vi "Scope_5761.vi"() -> ()   [LabVIEW 2013]
uses:
  <vilib>/userdefined/High Color/nirio_resource_hc.ctl
  FPGA/DataMode.ctl
  <vilib>/Analysis/4window.llb/windowTd.ctl
  Host/Scope/controls/power_spectrum_unit.ctl
  Host/Scope5782/Scope/controls/5782_trigger_type.ctl
  Host/Scope/controls/Data_calc_mode.ctl
  Host/Scope/controls/Data_display_mode.ctl
  Host/Scope/controls/Graph_references.ctl
  Host/Scope/controls/graph_controls.ctl
  Host/Scope/controls/Channel_select.ctl
  Host/Communication/Driver/RemoteConnection/RemoteConnection.lvclass
  Host/FpgaRef/FpgaRef5761/ClockSource_5761.ctl
  Host/Scope/Scope5671/Scope5761.lvclass
  Host/Scope/ScopeBase/ScopeBase.lvclass/ScopeBase.ctl
  FPGA/fpga_settings.ctl
  Host/Scope/controls/ScopeMode.ctl
  Host/Communication/global_stop.vi
  <vilib>/FPGAPlugInAG/PXIe-7975R/niLvFpga_Open_PXIe-7975R.vi
  <vilib>/rvi/interface/common/dynamic/niFpgaDynamicAddResources.vi
  <vilib>/rvi/interface/nirviOpenFPGA/nirviOpenFPGA.xnode
  FPGA Bitfiles/FPGAmain_5761_zPCTJJmozx4.lvbitx
  FPGAmain_5761.vi
  FPGA Bitfiles/FPGAmain5782_W462Q9ePIkg.lvbitx
  <vilib>/rvi/FXPMathLib/FxpInterpret/XNode/nifxpmath_Interpret.xnode
  Host/FpgaRef/FpgaRef5761/FpgaRef5761.lvclass
  Host/Scope/ScopeBase/ScopeBase.lvclass
  Host/FpgaRef/FpgaRef5782/FpgaRef5782.lvclass
  <vilib>/Analysis/NI_AALPro.lvlib
panel:
  in  "5761 -1  resource 2":T1="RIO0"
  in  "5761 -1  resource":T1="RIO0"
  in  "Ch3":bool
  in  "Ch2":bool
  in  "Ch1":bool
  in  "Ch0":bool
  in  "Ch3":bool
  in  "Ch2":bool
  in  "Ch1":bool
  in  "Ch0":bool
  in  "Ch3 Q":bool
  in  "Ch3 I":bool
  in  "Ch2 Q":bool
  in  "Ch2 I":bool
  in  "Ch1 Q":bool
  in  "Ch1 I":bool
  in  "Ch0 Q":bool
  in  "Ch0 I":bool
  in  "Ch3 Q":bool
  in  "Ch3 I":bool
  in  "Ch2 Q":bool
  in  "Ch2 I":bool
  in  "Ch1 Q":bool
  in  "Ch1 I":bool
  in  "Ch0 Q":bool
  in  "Ch0 I":bool
  in  "deltaF":bool
  in  "#bins":i32=1 min=1 max=16
  in  "ch1 DC offset":dbl caption="DC offset\nChannel 1"
  in  "ch0 DC offset":dbl caption="DC offset\nChannel 0"
  in  "Chart length":i32=200000
  in  "Trigmode":enum32{"Triggered", "Continuous"}(radio)
  in  "Refence for phase":T2
  in  "Graph_refs":T3
  out "Lower chart":dbl[][](graph)
  out "Upper chart":dbl[][](graph)
  out "Lower graph":i16[][](graph)
  in  "Buffer":T5
  in  "Display":T6
  in  "Trigger":T7
  in  "Ch1 Q":bool
  in  "Ch1 I":bool
  in  "Ch0 Q":bool
  in  "Ch0 I":bool
  in  "Ch1":bool
  in  "Ch0":bool
  out "stop 2":bool
  in  "Zoom freq X":bool
  in  "Zoom freq Y":bool
  in  "Zoom time Y":bool
  in  "Zoom time X":bool
  in  "Unit":T8
  in  "Window":T9=1 items=["Rectangle"=0, "Hanning"=1, "Hamming"=2, "Blackman-Harris"=3, "Exact Blackman"=4, "Blackman"=5, "Flat Top"=6, "4 Term B-Harris "=7, "7 Term B-Harris"=8, "Low Sidelobe"=9, "Blackman Nuttall"=11, "Triangle"=30, "Bartlett-Hanning"=31, "Bohman"=32, "Parzen"=33, "Welch"=34, "Kaiser"=60, "Dolph-Chebyshev"=61, "Gaussian"=62]
  in  "Samples per 5782 record":i32
  in  "Phase offset (deg)":dbl
  in  "Fequency [MHz]":dbl format="%#_8g"
  in  "Mode":T10
  in  "Mixer freq [MHz]":dbl
  out "freqdata":cluster{"f0":dbl, "df":dbl, "magnitude":dbl[]}[](graph)
  in  "Rumode":bool
  in  "Singleshot":bool
  out "error IO":errorcluster
  in  "stop":bool
  in  "resource name":T1="RIO0"
  # "5161 - 1"
  # "5161 - 2"
  # "FPGA setup"
  # "V"
  # "V"
  # "Auto Zoom"
  # "5782"
  # "5161 - 1"
  # "Simulated data"
  # "5161 - 2"
  # "FFT"
  # "Auto Zoom"
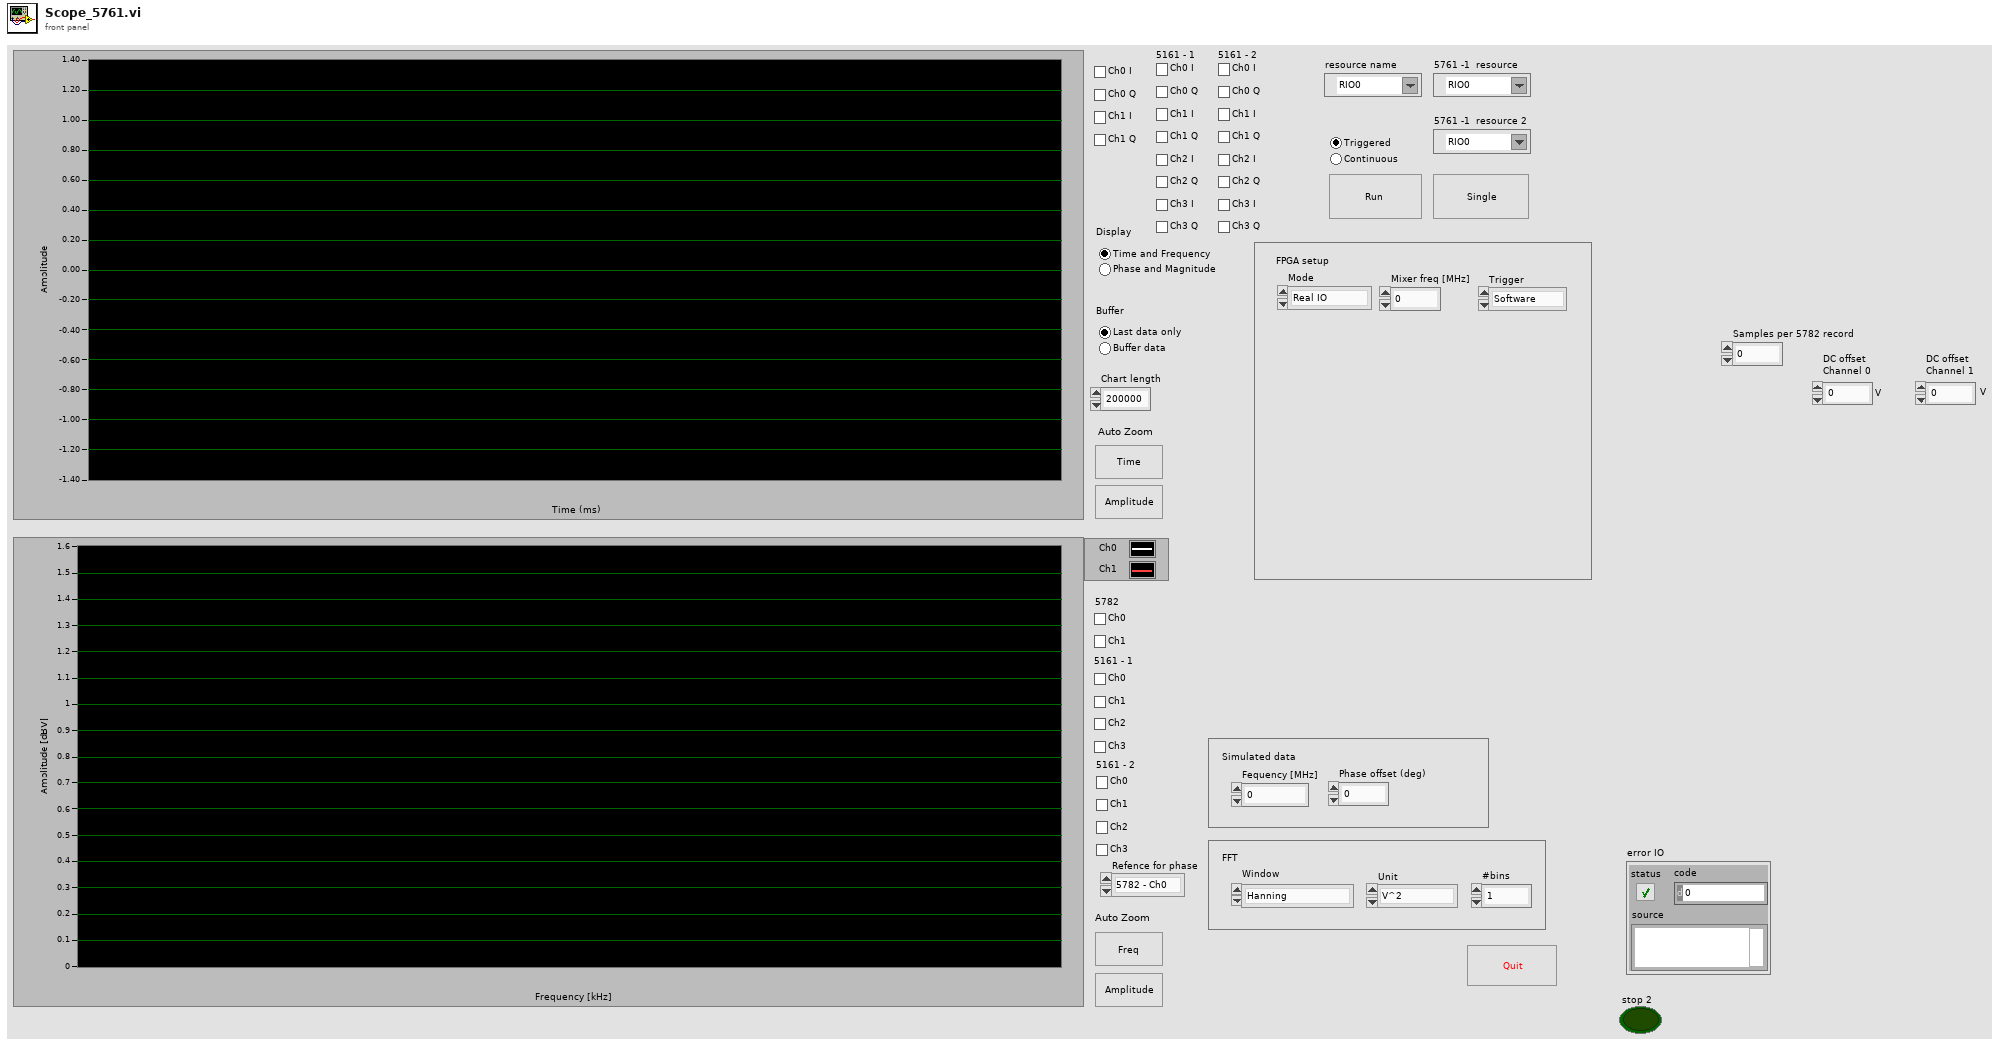
[diagram p1: front panel]
types:
  T1 = typedef "nirio_resource_hc.ctl" = tag
  T2 = typedef "Channel_select.ctl" = enum16{"5782 - Ch0", "5782 - Ch1"}
  T3 = typedef "Graph_references.ctl" = cluster{"upper":T4, "lower":T4, "Freq graph":refnum<vi>}
  T4 = typedef "graph_controls.ctl" = cluster{"Graph":refnum<vi>, "Time btn":refnum<vi>, "Amplitude btn":refnum<vi>, "Chart":refnum<vi>}
  T5 = typedef "Data_display_mode.ctl" = enum32{"Last data only", "Buffer data"}
  T6 = typedef "Data_calc_mode.ctl" = enum32{"Time and Frequency", "Phase and Magnitude"}
  T7 = typedef "5782_trigger_type.ctl" = enum16{"Software", "Trigger input"}
  T8 = typedef "power_spectrum_unit.ctl" = enum16{"V^2", "V", "dBV"}
  T9 = typedef "NI_AALPro.lvlib/windowTd.ctl" = u32
  T10 = typedef "DataMode.ctl" = enum16{"Real IO", "Simulated"}
  T11 = typedef "ClockSource_5761.ctl" = enum8{"Internal Clock PLL Off", "Internal Clock PLL On (CLK_IN)", "External Clock (CLK_IN)", "Internal Clock PLL On (IoModSyncClk)", "External Clock (IoModSyncClk)"}
  T12 = enum8{"Internal Clock PLL Off", "Internal Clock PLL On (REF IN)", "External Clock (CLK_IN)", "Internal Clock PLL On (IoModSyncClk)"}
  T13 = typedef "fpga_settings.ctl" = enum16{"Feedback Enable", "New FIR coeffs", "FIR shift", "Enable filter", "Set Downsample", "Downsample", "CIC Gain", "Record length", "Trigger samples", "Quiet time", "a_am", "b_am", "Use fixed delay", "fixed sin_fi", "fixed cos_fi", "Ki*Tau", "Kp", "Kd_Tau", "Fi_start", "Fi_delta", "DC_offs 0", "DC_offs 1", "Ki*Tau am", "Kp am", "Kd_Tau am", "Feedback AM"}
  T14 = typedef "ScopeMode.ctl" = enum16{"Stopped", "Single", "Running", "Continuous"}
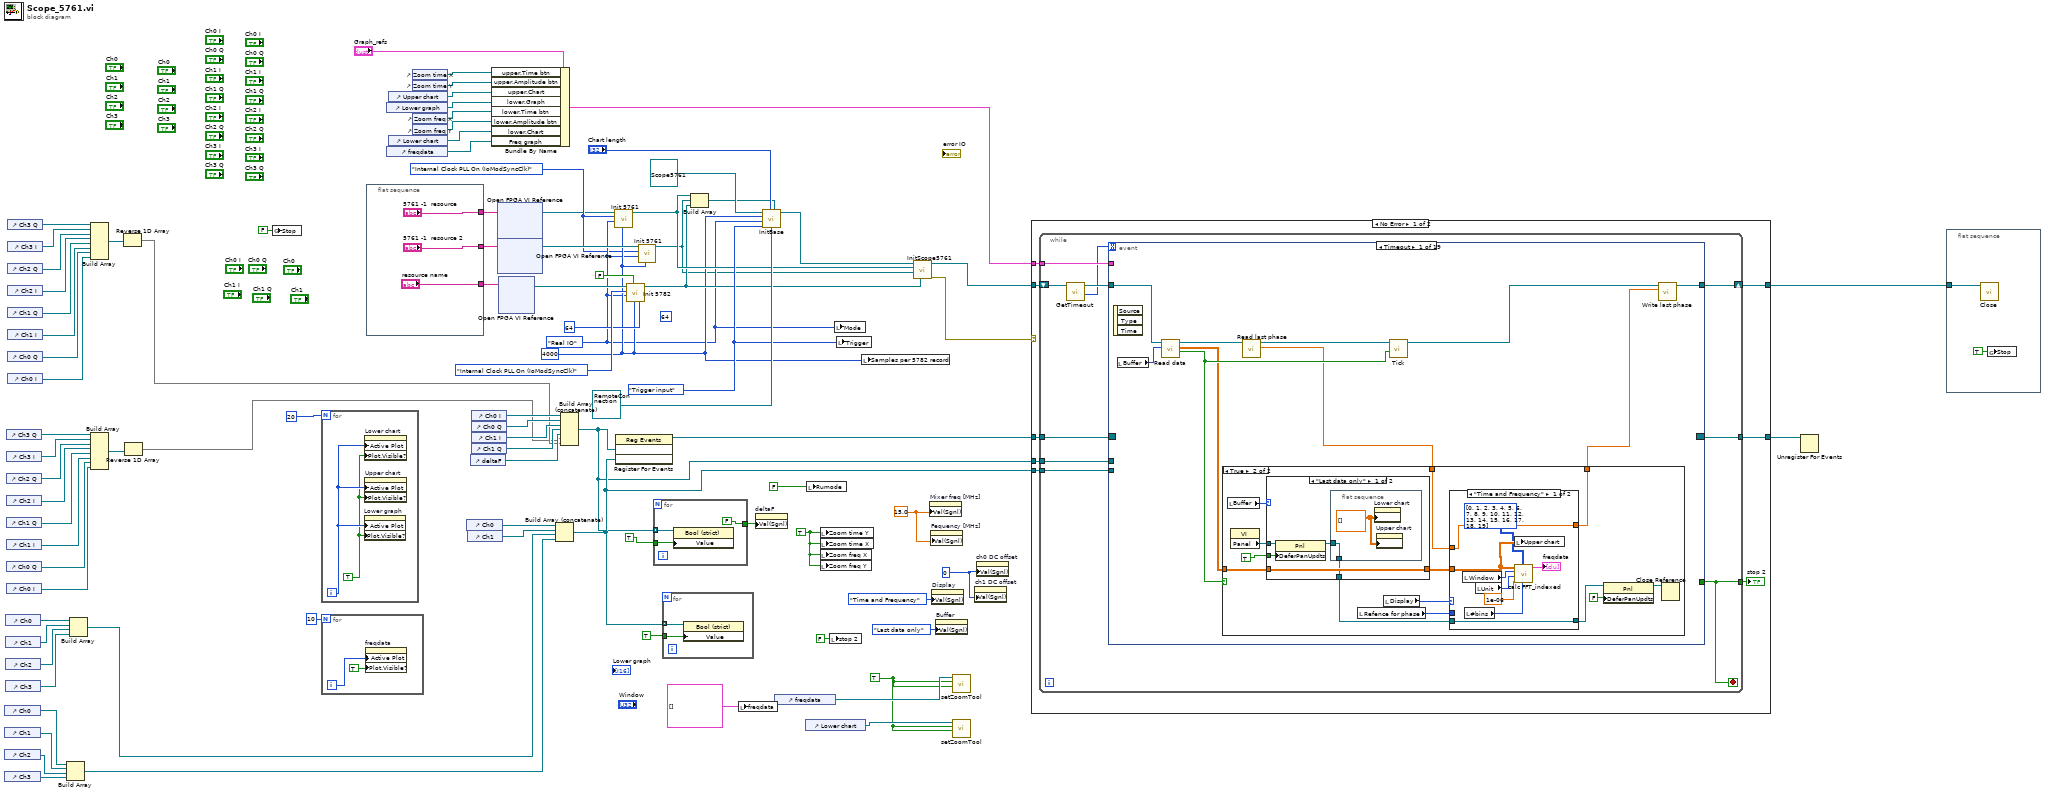
[diagram p0: block diagram]
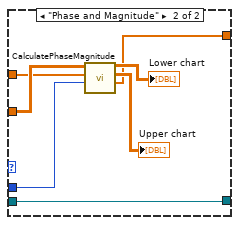
[diagram p4: hidden frame]
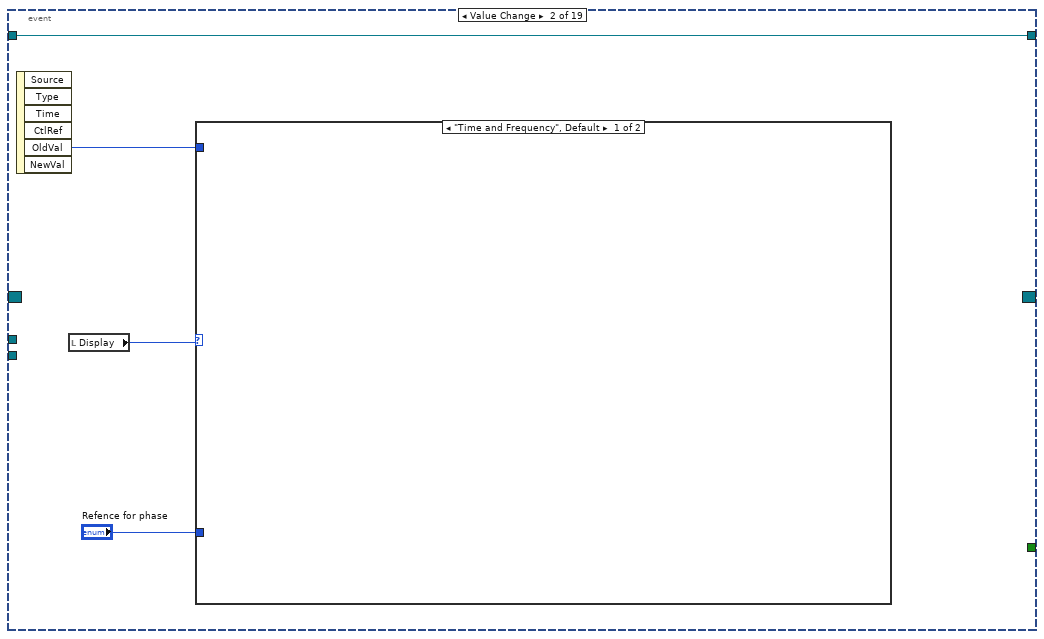
[diagram p5: hidden frame]
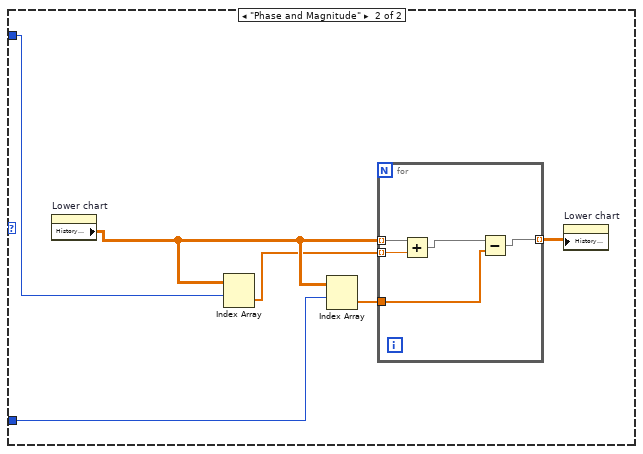
[diagram p6: hidden frame]
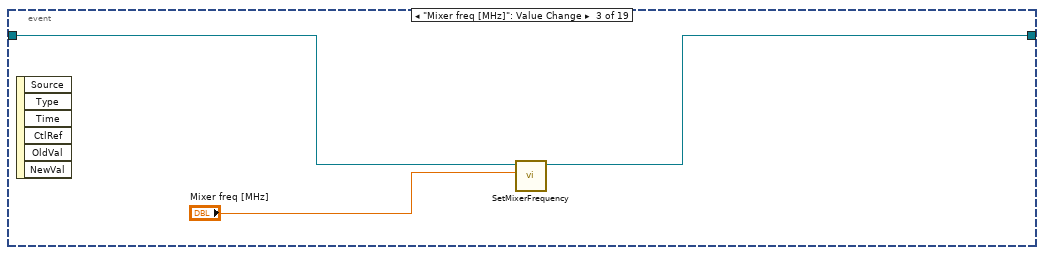
[diagram p7: hidden frame]
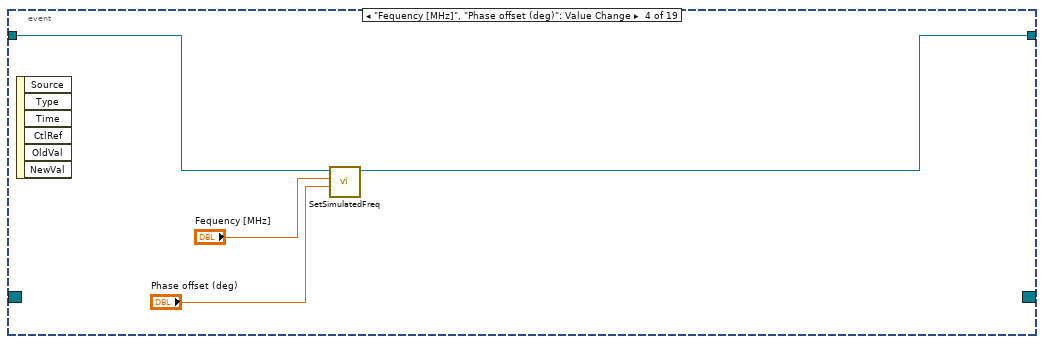
[diagram p8: hidden frame]
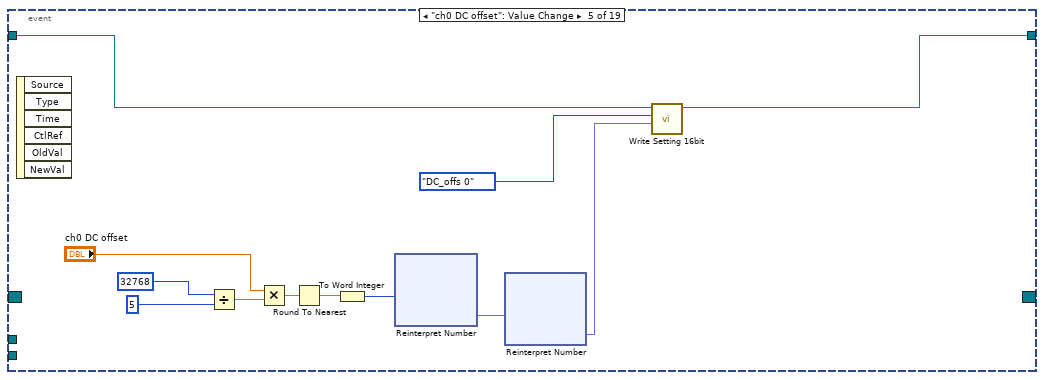
[diagram p9: hidden frame]
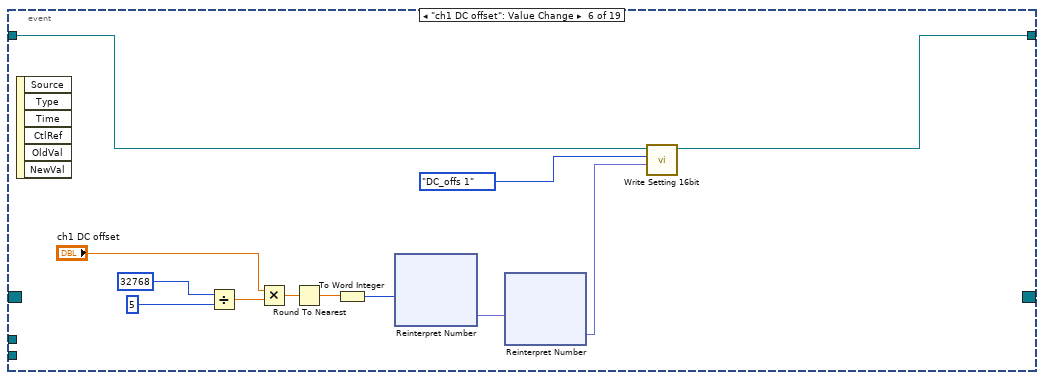
[diagram p10: hidden frame]
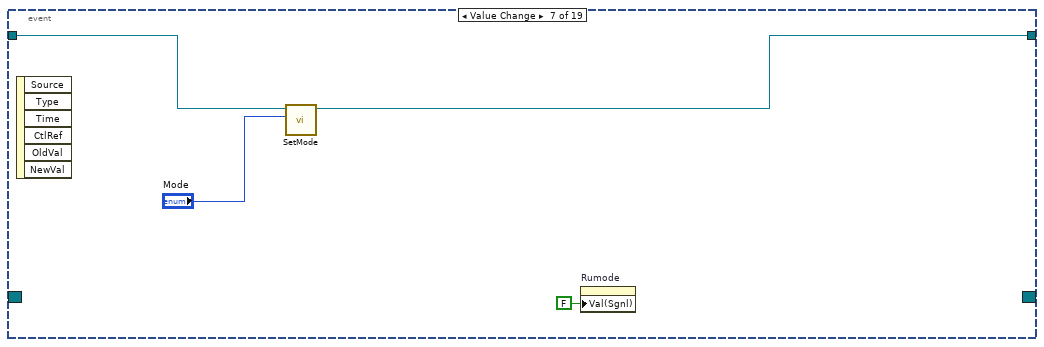
[diagram p11: hidden frame]
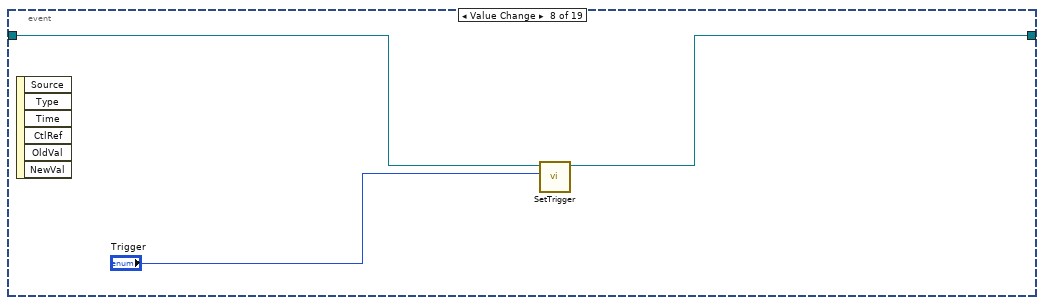
[diagram p12: hidden frame]
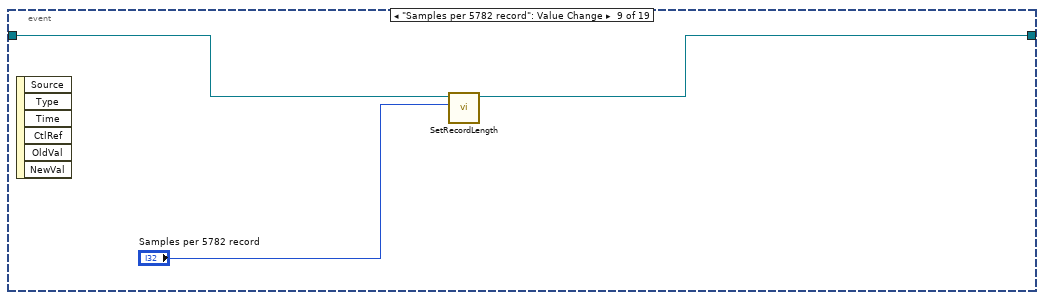
[diagram p13: hidden frame]
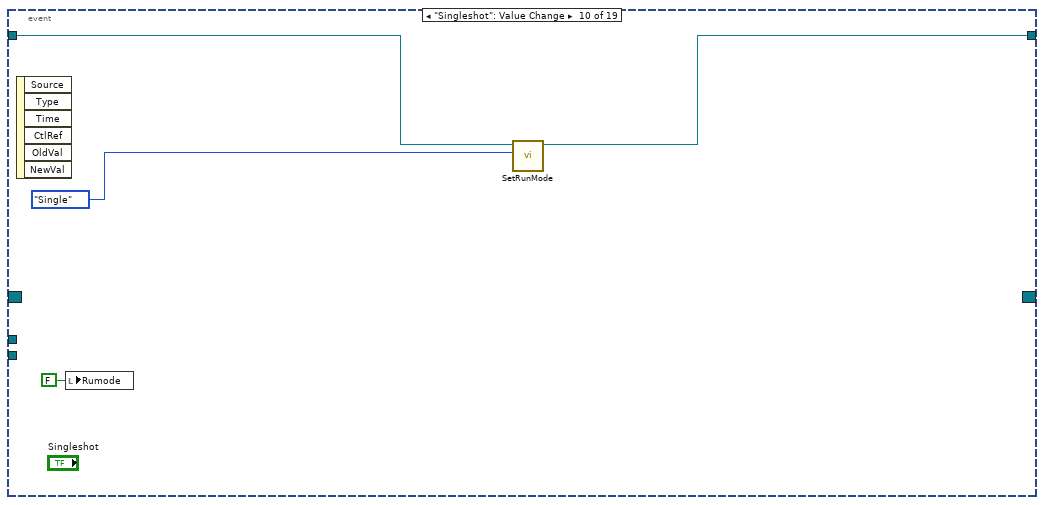
[diagram p14: hidden frame]
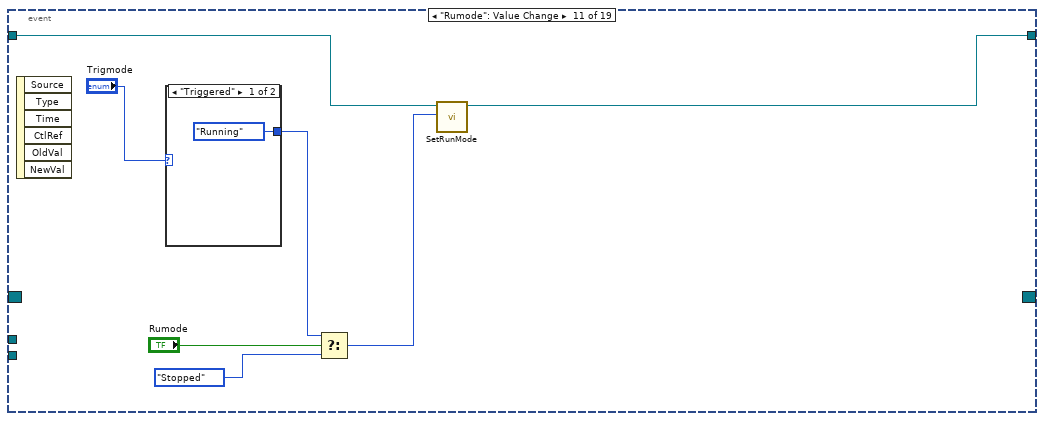
[diagram p15: hidden frame]
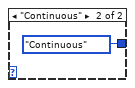
[diagram p16: hidden frame]
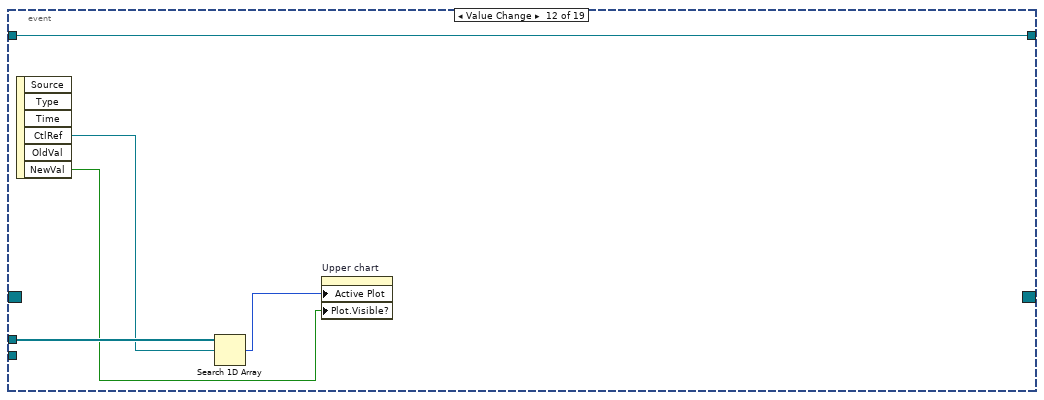
[diagram p17: hidden frame]
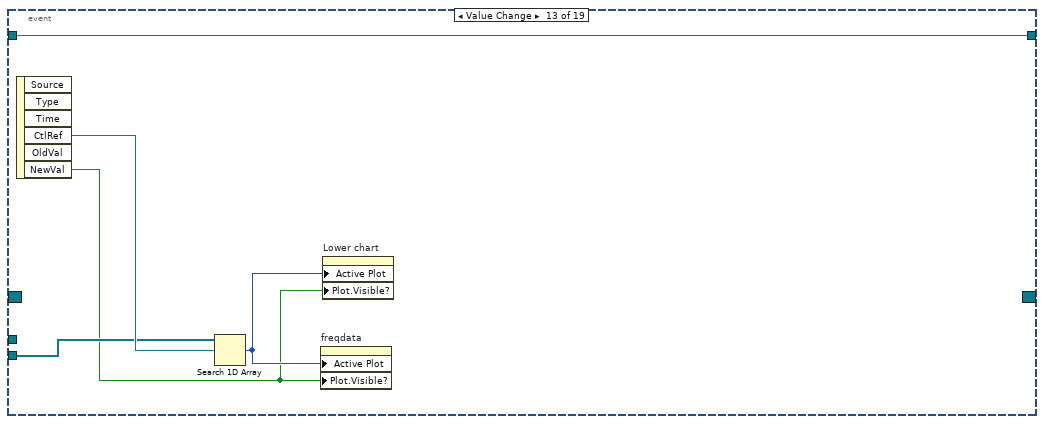
[diagram p18: hidden frame]
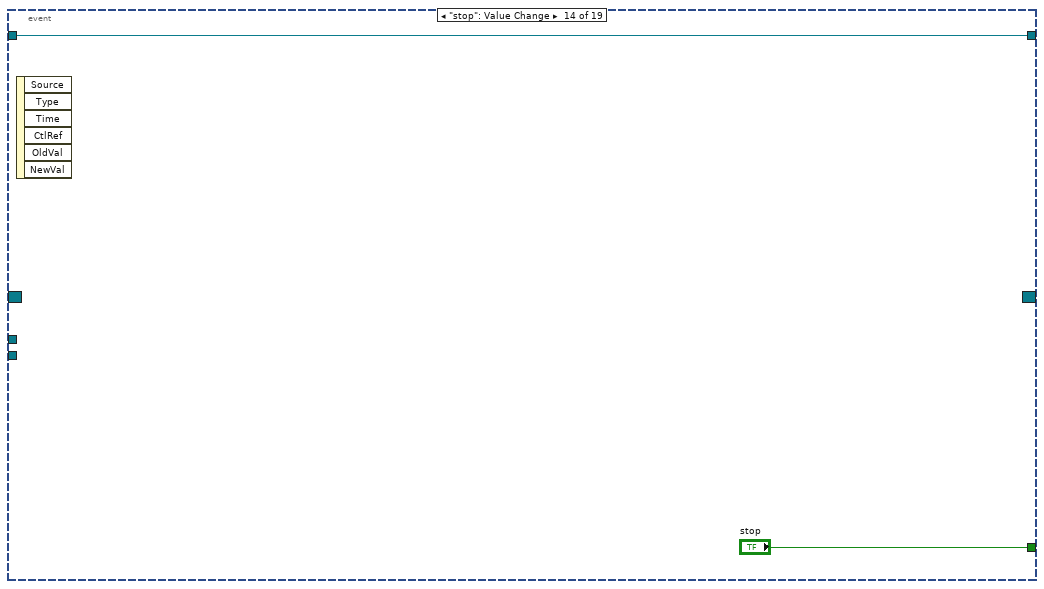
[diagram p19: hidden frame]
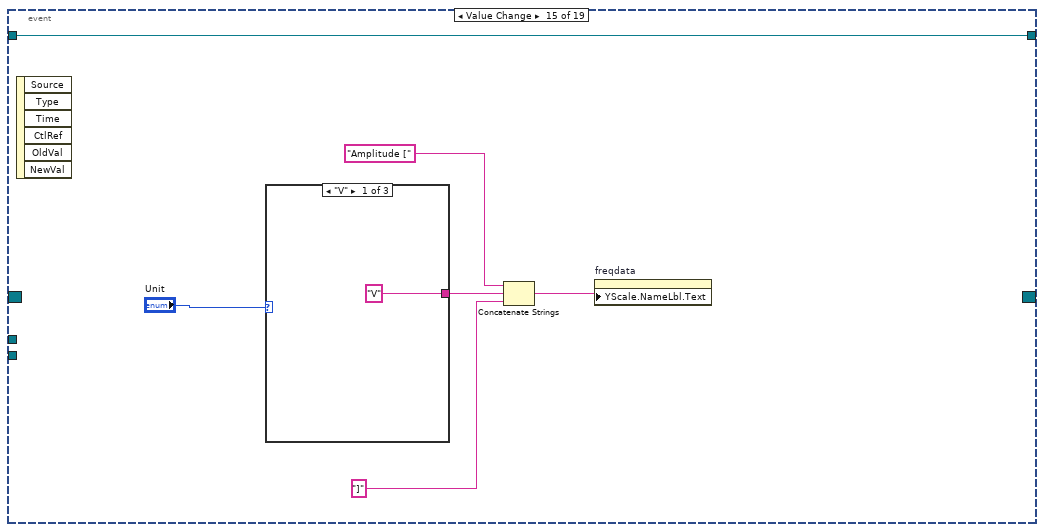
[diagram p20: hidden frame]
diagram:
  w4 = ClockSource_5761."Internal Clock PLL On (IoModSyncClk)" ("Clock Source")
  (unwired) u8 64 ("User Data 1")
  w60 = i16 0 ("Value (Signaling)")
  w21 = 5782_trigger_type."Trigger input" ("Trigger")
  w57 = TRUE ("Zoom  X")
  w54 = TRUE ("Rumode")
  w5 = DataMode."Real IO" ("Mode")
  w6 = u16 4000 ("Samples to aqcuire")
  w90 = 15.0 ("Mixer requency [MHz]")
  n1 = control-ref of="Ch0"() -> (w30:refnum<vi>)
  n2 = control-ref of="Ch1"() -> (w31:refnum<vi>)
  n3 = control-ref of="Ch2"() -> (w32:refnum<vi>)
  n4 = control-ref of="Ch3"() -> (w33:refnum<vi>)
  n5 = control-ref of="Ch0"() -> (w29:refnum<vi>)
  n6 = control-ref of="Ch1"() -> (w28:refnum<vi>)
  n7 = control-ref of="Ch2"() -> (w27:refnum<vi>)
  n8 = control-ref of="Ch3"() -> (w26:refnum<vi>)
  n9 = control-ref of="Ch3 Q"() -> (w45:refnum<vi>)
  n10 = control-ref of="Ch3 I"() -> (w44:refnum<vi>)
  n11 = control-ref of="Ch2 Q"() -> (w43:refnum<vi>)
  n12 = control-ref of="Ch2 I"() -> (w42:refnum<vi>)
  n13 = control-ref of="Ch1 Q"() -> (w37:refnum<vi>)
  n14 = control-ref of="Ch1 I"() -> (w36:refnum<vi>)
  n15 = control-ref of="Ch0 Q"() -> (w34:refnum<vi>)
  n16 = control-ref of="Ch0 I"() -> (w35:refnum<vi>)
  n17 = control-ref of="Ch3 Q"() -> (w53:refnum<vi>)
  n18 = control-ref of="Ch3 I"() -> (w52:refnum<vi>)
  n19 = control-ref of="Ch2 Q"() -> (w51:refnum<vi>)
  n20 = control-ref of="Ch2 I"() -> (w50:refnum<vi>)
  n21 = control-ref of="Ch1 Q"() -> (w49:refnum<vi>)
  n22 = control-ref of="Ch1 I"() -> (w48:refnum<vi>)
  n23 = control-ref of="Ch0 Q"() -> (w47:refnum<vi>)
  n24 = control-ref of="Ch0 I"() -> (w46:refnum<vi>)
  n25 = Build Array(w30, w31, w32, w33) -> (w25:refnum<vi>[])
  n26 = Build Array(w29, w28, w27, w26) -> (w24:refnum<vi>[])
  n27 = Build Array(w53, w52, w51, w50, w49, w48, w47, w46) -> (w41:refnum<vi>[])
  n28 = Build Array(w45, w44, w43, w42, w37, w36, w34, w35) -> (w40:refnum<vi>[])
  n29 = Reverse 1D Array(array=w41) -> (reversed array=w39:refnum<vi>[])
  n30 = Reverse 1D Array(array=w40) -> (reversed array=w38:refnum<vi>[])
  n31 = global write "global_stop.vi" "Stop"(FALSE ("Stop")) -> ()
  n32 = for {
    N: 20 -> [_]
    i -> [w94]
    w93 = TRUE ("Plot.Visible")
    n33 = property on="Lower graph" class="WFGraph (strict)"("Active Plot"=w94, "Plot.Visible?"=w93) -> ()  [unwired: 2 in, 2 out]
    n34 = property on="Lower chart" class="WFChart (strict)"("Active Plot"=w94, "Plot.Visible?"=w93) -> ()  [unwired: 2 in, 2 out]
    n35 = property on="Upper chart" class="WFChart (strict)"("Active Plot"=w94, "Plot.Visible?"=w93) -> ()  [unwired: 2 in, 2 out]
  }
  n36 = for {
    N: 10 -> [_]
    i -> [w95]
    n37 = property on="freqdata" class="WFGraph (strict)"("Active Plot"=w95, "Plot.Visible?"=TRUE ("Plot.Visible")) -> ()  [unwired: 2 in, 2 out]
  }
  n38 = flat-sequence {
    tunnel: ["resource name"] -> w82
    tunnel: ["5761 -1  resource"] -> w23
    tunnel: ["5761 -1  resource 2"] -> w7
    frame #0 {
    }
  }
  n39 = control-ref of="Lower graph"() -> (w68:refnum<vi>)
  n40 = control-ref of="freqdata"() -> (w64:refnum<vi>)
  n41 = control-ref of="Upper chart"() -> (w69:refnum<vi>)
  n42 = control-ref of="Lower chart"() -> (w65:refnum<vi>)
  n43 = control-ref of="Zoom time X"() -> (w71:refnum<vi>)
  n44 = control-ref of="Zoom time Y"() -> (w70:refnum<vi>)
  n45 = control-ref of="Zoom freq X"() -> (w67:refnum<vi>)
  n46 = control-ref of="Zoom freq Y"() -> (w66:refnum<vi>)
  n47 = control-ref of="Ch0"() -> (w79:refnum<vi>)
  n48 = control-ref of="Ch1"() -> (w80:refnum<vi>)
  n49 = control-ref of="deltaF"() -> (w55:refnum<vi>)
  n50 = control-ref of="Ch0 I"() -> (w75:refnum<vi>)
  n51 = control-ref of="Ch0 Q"() -> (w76:refnum<vi>)
  n52 = control-ref of="Ch1 I"() -> (w77:refnum<vi>)
  n53 = control-ref of="Ch1 Q"() -> (w78:refnum<vi>)
  n54 = Bundle By Name(cluster="Graph_refs", "upper.Time btn"=w71, "upper.Amplitude btn"=w70, "upper.Chart"=w69, "lower.Graph"=w68, "lower.Time btn"=w67, "lower.Amplitude btn"=w66, "lower.Chart"=w65, "Freq graph"=w64) -> (w63:T3)
  n55 = xnode "Open FPGA VI Reference"("resource name"=w23) -> ("FPGA VI Reference Out"=w2:refnum<k20>)  [unwired: 1 in, 1 out]
  n56 = xnode "Open FPGA VI Reference"("resource name"=w7) -> ("FPGA VI Reference Out"=w8:refnum<k20>)  [unwired: 1 in, 1 out]
  n57 = xnode "Open FPGA VI Reference"("resource name"=w82) -> ("FPGA VI Reference Out"=w17:refnum<k20>)  [unwired: 1 in, 1 out]
  n58 = Build Array (concatenate)(w79, w80, w24, w25) -> (w83:refnum<vi>[])
  n59 = Build Array (concatenate)(w75, w76, w77, w78, w55, w38, w39) -> (w74:refnum<vi>[])
  n60 = call "Init 5761.vi"("Record length"=w6, "Mode"=w5, "Clock Source"=w4, "FPGA ref"=w2) -> ("FpgaRef5761 out"=w13:refnum<class "FpgaRef5761.lvclass">)  [unwired: 6 in, 1 out]
  n61 = register-events(w74, w83) -> (reference out=w87:refnum<event-registration>)  [unwired: 2 in, 1 out]
  n62 = call "Init 5782.vi"("User Data 1"=u8 64, "Record length"=w6, "Use 1Mhz clock"=FALSE, "Mode"=w5, "Clock Source"=T12."Internal Clock PLL On (IoModSyncClk)", "FPGA ref"=w17) -> ("FpgaRef5782 Out"=w11:refnum<class "FpgaRef5782.lvclass">)  [unwired: 4 in, 1 out]
  n63 = call "Init 5761.vi"("Record length"=w6, "Mode"=w5, "Clock Source"=w4, "FPGA ref"=w8) -> ("FpgaRef5761 out"=w3:refnum<class "FpgaRef5761.lvclass">)  [unwired: 6 in, 1 out]
  n64 = for {
    tunnel: w74 -> [w102] mode=indexing
    tunnel: TRUE ("Rumode") -> [w101]
    tunnel: [FALSE ("Rumode")] -> w56
    n65 = property class="Bool (strict)"(reference=w102, "Value"=w101) -> ()  [unwired: 1 in, 2 out]
  }
  n66 = for {
    tunnel: w83 -> [w104] mode=indexing
    tunnel: TRUE ("Rumode") -> [w103]
    n67 = property class="Bool (strict)"(reference=w104, "Value"=w103) -> ()  [unwired: 1 in, 2 out]
  }
  n68 = Build Array(w13, w3, w11) -> (w12:refnum<class "FpgaRefBase.lvclass">[])
  n69 = local write "freqdata"(cluster{"f0":dbl, "df":dbl, "magnitude":dbl[]}[] [] ("freqdata")) -> ()
  n70 = property on="deltaF" class="Bool (strict)"("Val(Sgnl)"=w56) -> ()  [unwired: 2 in, 2 out]
  n71 = call "InitBase.vi"("FPGA refs"=w12, "RemoteConnection"=refnum<class "RemoteConnection.lvclass"> refnum, "Chart length"="Chart length", "Trigger"=w21, "data mode"=w5, "Samples Per Trigger"=w6, "ScopeBase in"=refnum<class "Scope5761.lvclass"> refnum ("Scope5761 out")) -> ("ScopeBase out"=w19:refnum<class "Scope5761.lvclass">)  [unwired: 4 in]
  n72 = control-ref of="freqdata"() -> (w73:refnum<vi>)
  n73 = control-ref of="Lower chart"() -> (w58:refnum<vi>)
  n74 = local write "Rumode"(FALSE ("Rumode")) -> ()
  n75 = local write "Zoom time Y"(w54) -> ()
  n76 = local write "Zoom time X"(w54) -> ()
  n77 = local write "Zoom freq X"(w54) -> ()
  n78 = local write "Zoom freq Y"(w54) -> ()
  n79 = local write "stop 2"(FALSE ("stop 2")) -> ()
  n80 = local write "Mode"(w5) -> ()
  n81 = local write "Trigger"(w21) -> ()
  n82 = local write "Samples per 5782 record"(w6) -> ()
  n83 = call "InitScope5761.vi"("FpgaRef5782"=w11, "FpgaRef5761 - 2"=w3, "FpgaRef5761 - 1"=w13, "Scope5761 in"=w19) -> ("error out"=w9:errorcluster, "Scope5761 out"=w10:refnum<class "Scope5761.lvclass">)  [unwired: 6 in]
  n84 = property on="Mixer freq [MHz]" class="DigNum (strict)"("Val(Sgnl)"=w90) -> ()  [unwired: 2 in, 2 out]
  n85 = property on="Fequency [MHz]" class="DigNum (strict)"("Val(Sgnl)"=w90) -> ()  [unwired: 2 in, 2 out]
  n86 = property on="Display" class="RadioBtnsControl (strict)"("Val(Sgnl)"=Data_calc_mode."Time and Frequency" ("Value (Signaling)")) -> ()  [unwired: 2 in, 2 out]
  n87 = property on="Buffer" class="RadioBtnsControl (strict)"("Val(Sgnl)"=enum32{"Last data only", "Buffer data"}."Last data only" ("Value (Signaling)")) -> ()  [unwired: 2 in, 2 out]
  n88 = call "setZoomTool.vi"("Zoom Y"=w57, "Zoom  X"=w57, "reference"=w58) -> ()  [unwired: 9 in]
  n89 = call "setZoomTool.vi"("Zoom Y"=w57, "Zoom  X"=w57, "reference"=w73) -> ()  [unwired: 9 in]
  n90 = property on="ch1 DC offset" class="DigNum (strict)"("Val(Sgnl)"=w60) -> ()  [unwired: 2 in, 2 out]
  n91 = property on="ch0 DC offset" class="DigNum (strict)"("Val(Sgnl)"=w60) -> ()  [unwired: 2 in, 2 out]
  n92 = case shown="No Error" w9 {
    tunnel: w10 -> [w112 w292]
    tunnel: [w111 w292] -> w1
    tunnel: w87 -> [w110 w291]
    tunnel: [w109 w291] -> w86
    tunnel: w74 -> [w108 _]
    tunnel: w83 -> [w107 _]
    tunnel: w63 -> [w105 _]
    frame No Error {
      n93 = while {
        shift-right: [w122] -> w111
        shift-left: w112 -> [w115]
        tunnel: w110 -> [w121]
        tunnel: [w120] -> w109
        tunnel: w108 -> [w119]
        tunnel: w107 -> [w118]
        tunnel: [w117] -> w106
        tunnel: w105 -> [w116]
        stop <- w117 stop-if-true
        n94 = call "GetTimeout.vi"("ScopeBase in"=w115) -> ("Time left"=w113:i32, "ScopeBase out"=w114:refnum<class "Scope5761.lvclass">)  [unwired: 8 in, 1 out]
        n95 = event shown="[0] Timeout" {
          selector: w121 -> [_ _ _ _ _ _ _ _ _ _ _ _ _ _ _ _ _ _ _]
          dyn-events: [_ _ _ _ _ _ _ _ _ _ _ _ _ _ _ _ _ _ _] -> w120
          timeout: w113 -> [_ _ _ _ _ _ _ _ _ _ _ _ _ _ _ _ _ _ _]
          tunnel: [_ _ _ _ _ _ _ _ _ _ _ _ _ "stop" _ _ _ _ _] -> w117
          tunnel: w114 -> [w129 w175 w189 w191 w195 w207 w220 w223 w227 w230 w234 w245 w250 w251 w258 w268 w272 w278 w281]
          tunnel: [w132 w175 w187 w190 w194 w206 w218 w222 w225 w228 w232 w245 w250 w251 w258 w268 w272 w278 w279] -> w122
          tunnel: w119 -> [_ _ _ _ _ _ _ _ _ _ _ w244 _ _ _ _ _ _ _]
          tunnel: w118 -> [_ _ _ _ _ _ _ _ _ _ _ _ w248 _ _ _ _ _ _]
          tunnel: w116 -> [_ _ _ _ _ _ _ _ _ _ _ _ _ _ _ _ _ _ w288]
          event Timeout {
            n96 = event-data() -> ()  [unwired: 1 in, 3 out]
            n97 = local read "Buffer"() -> (w128:T5)
            n98 = call-dynamic "Read data.vi"("Buffer mode"=w128, "Scope5761 in"=w129) -> ("Any read?"=w127:bool, "Data"=w126:dbl[][], "Scope5761 out"=w124:refnum<class "Scope5761.lvclass">)  [unwired: 6 in, 1 out]
            n99 = call "Read last phase.vi"("ScopeBase in"=w124) -> ("last phase"=w125:dbl[], "ScopeBase out"=w123:refnum<class "Scope5761.lvclass">)  [unwired: 8 in, 1 out]
            n100 = case shown="True" w127 {
              tunnel: w126 -> [_ w143]
              tunnel: w125 -> [w133 w135]
              tunnel: [w133 w134] -> w131
              frame False {
              }
              frame True {
                n101 = local read "Buffer"() -> (w145:T5)
                n102 = property class="VI"() -> ("Panel"=w138:refnum<vi>)  [unwired: 2 in, 2 out]
                n103 = case shown="\"Last data only\"" w145 {
                  tunnel: w143 -> [w151 w155]
                  tunnel: [w151 w155] -> w144
                  tunnel: w138 -> [w150 w154]
                  tunnel: TRUE ("Defer Panel Updates") -> [w148 _]
                  tunnel: [w147 w154] -> w136
                  frame "Last data only" {
                    n104 = property class="Pnl"(reference=w150, "DeferPanUpdts"=w148) -> (reference out=w149:refnum<vi>)  [unwired: 1 in, 1 out]
                    n105 = flat-sequence {
                      tunnel: w149 -> [w152]
                      tunnel: [w152] -> w147
                      frame #0 {
                        w153 = dbl[][] [] ("History Data")
                        n106 = property on="Lower chart" class="WFChart (strict)"("History Data"=w153) -> ()  [unwired: 2 in, 2 out]
                        n107 = property on="Upper chart" class="WFChart (strict)"("History Data"=w153) -> ()  [unwired: 2 in, 2 out]
                      }
                    }
                  }
                  frame "Buffer data" {
                  }
                }
                n108 = local read "Refence for phase"() -> (w142:T2)
                n109 = local read "Display"() -> (w146:T6)
                n110 = case shown="\"Time and Frequency\"" w146 {
                  tunnel: w144 -> [w160 w171]
                  tunnel: w142 -> [_ w168]
                  tunnel: [w159 w167] -> w140
                  tunnel: w136 -> [w159 w167]
                  tunnel: w135 -> [w157 w166]
                  tunnel: [w157 w165] -> w134
                  frame "Time and Frequency" {
                    n111 = local read "Window"() -> (w161:T9)
                    n112 = local read "#bins"() -> (w158:i32)
                    n113 = local read "Unit"() -> (w162:T8)
                    n114 = local write "Upper chart"(w160) -> ()
                    n115 = call "calc FFT_indexed.vi"("#bins"=w158, "IQ indexes"=i32[][] [[0, 1], [2, 3], [4, 5], [6, 7], [8, 9], [10, 11], [12, 13], [14, 15], [16, 17], [18, 19]], "dt"=1e-06, "Unit"=w162, "Window"=w161, "data"=w160) -> ("Power Spectrum / PSD"=→"freqdata":cluster{"f0":dbl, "df":dbl, "magnitude":dbl[]}[])  [unwired: 5 in]
                  }
                  frame "Phase and Magnitude" {
                    n116 = call "CalculatePhaseMagnitude.vi"("phase reference channel"=w168, "previous phase"=w166, "data"=w171) -> ("last phase"=w165:dbl[], "Magnitude"=→"Upper chart":dbl[][], "Phase"=→"Lower chart":dbl[][])  [unwired: 6 in]
                  }
                }
                n117 = property class="Pnl"(reference=w140, "DeferPanUpdts"=FALSE ("Defer Panel Updates")) -> (reference out=w139:refnum<vi>)  [unwired: 1 in, 1 out]
                n118 = Close Reference(reference=w139) -> ()  [unwired: 1 in, 1 out]
              }
            }
            n119 = call "Tick.vi"("Any elements read?"=w127, "ScopeBase in"=w123) -> ("ScopeBase out"=w130:refnum<class "Scope5761.lvclass">)  [unwired: 8 in, 1 out]
            n120 = call "Write last phase.vi"("last phase"=w131, "ScopeBase in"=w130) -> ("ScopeBase out"=w132:refnum<class "Scope5761.lvclass">)  [unwired: 8 in, 1 out]
          }
          event Value Change {
            n121 = event-data() -> ("OldVal"=w172:T2)  [unwired: 1 in, 5 out]
            n122 = local read "Display"() -> (w173:T6)
            n123 = case shown="\"Time and Frequency\", Default" w173 {
              tunnel: "Refence for phase" -> [_ w180]
              tunnel: w172 -> [_ w178]
              frame "Time and Frequency", Default {
              }
              frame "Phase and Magnitude" {
                n124 = property on="Lower chart" class="WFChart (strict)"() -> ("History Data"=w179:dbl[][])  [unwired: 2 in, 2 out]
                n125 = Index Array(array=w179, index (row)=w178) -> (element=w177:dbl[])  [unwired: 1 in]
                n126 = Index Array(array=w179, index (row)=w180) -> (element=w181:dbl[])  [unwired: 1 in]
                n127 = for {
                  tunnel: w179 -> [w184] mode=indexing
                  tunnel: w181 -> [w186]
                  tunnel: [w185] -> w176 mode=indexing
                  tunnel: w177 -> [w183] mode=indexing
                  n128 = Add(x=w184, y=w183) -> (x+y=w182:dbl[])
                  n129 = Subtract(x=w182, y=w186) -> (x-y=w185:dbl[])
                }
                n130 = property on="Lower chart" class="WFChart (strict)"("History Data"=w176) -> ()  [unwired: 2 in, 2 out]
              }
            }
          }
          event "Mixer freq [MHz]": Value Change {
            n131 = event-data() -> ()  [unwired: 1 in, 6 out]
            n132 = call-dynamic "SetMixerFrequency.vi"("Mixer freq [MHz]"="Mixer freq [MHz]", "ScopeBase In"=w189) -> ("ScopeBase Out"=w187:refnum<class "Scope5761.lvclass">)  [unwired: 8 in, 1 out]
          }
          event "Fequency [MHz]", "Phase offset (deg)": Value Change {
            n133 = event-data() -> ()  [unwired: 1 in, 6 out]
            n134 = call-dynamic "SetSimulatedFreq.vi"("Phase offset (deg)"="Phase offset (deg)", "Fequency [MHz]"="Fequency [MHz]", "ScopeBase In"=w191) -> ("ScopeBase Out"=w190:refnum<class "Scope5761.lvclass">)  [unwired: 7 in, 1 out]
          }
          event "ch0 DC offset": Value Change {
            n135 = event-data() -> ()  [unwired: 1 in, 6 out]
            n136 = Divide(x=32768, y=5) -> (x/y=w203:dbl)
            n137 = Multiply(x="ch0 DC offset", y=w203) -> (x*y=w201:dbl)
            n138 = Round To Nearest(number=w201) -> (nearest integer value=w200:dbl)
            n139 = To Word Integer(number=w200) -> (16bit integer=w199:i16)
            n140 = xnode "Reinterpret Number"("x"=w199) -> ("y"=w198:fxp<+/-,16,14>)
            n141 = xnode "Reinterpret Number"("x"=w198) -> ("y"=w196:fxp<+,16,16>)
            n142 = call "Write Setting 16bit.vi"("value"=w196, "FPGA Setting"=fpga_settings."DC_offs 0", "ScopeBase in"=w195) -> ("ScopeBase out"=w194:refnum<class "Scope5761.lvclass">)  [unwired: 7 in, 1 out]
          }
          event "ch1 DC offset": Value Change {
            n143 = event-data() -> ()  [unwired: 1 in, 6 out]
            n144 = Divide(x=32768, y=5) -> (x/y=w215:dbl)
            n145 = Multiply(x="ch1 DC offset", y=w215) -> (x*y=w214:dbl)
            n146 = Round To Nearest(number=w214) -> (nearest integer value=w213:dbl)
            n147 = To Word Integer(number=w213) -> (16bit integer=w212:i16)
            n148 = xnode "Reinterpret Number"("x"=w212) -> ("y"=w211:fxp<+/-,16,14>)
            n149 = xnode "Reinterpret Number"("x"=w211) -> ("y"=w210:fxp<+,16,16>)
            n150 = call "Write Setting 16bit.vi"("value"=w210, "FPGA Setting"=fpga_settings."DC_offs 1", "ScopeBase in"=w207) -> ("ScopeBase out"=w206:refnum<class "Scope5761.lvclass">)  [unwired: 7 in, 1 out]
          }
          event Value Change {
            n151 = event-data() -> ()  [unwired: 1 in, 6 out]
            n152 = call-dynamic "SetMode.vi"("Mode"="Mode", "ScopeBase In"=w220) -> ("ScopeBase Out"=w218:refnum<class "Scope5761.lvclass">)  [unwired: 8 in, 1 out]
            n153 = property on="Rumode" class="Bool (strict)"("Val(Sgnl)"=FALSE ("Value (Signaling)")) -> ()  [unwired: 2 in, 2 out]
          }
          event Value Change {
            n154 = event-data() -> ()  [unwired: 1 in, 6 out]
            n155 = call-dynamic "SetTrigger.vi"("Trigger"="Trigger", "ScopeBase In"=w223) -> ("ScopeBase Out"=w222:refnum<class "Scope5761.lvclass">)  [unwired: 8 in, 1 out]
          }
          event "Samples per 5782 record": Value Change {
            n156 = event-data() -> ()  [unwired: 1 in, 6 out]
            n157 = call-dynamic "SetRecordLength.vi"("Samples per 5782 record"="Samples per 5782 record", "ScopeBase In"=w227) -> ("ScopeBase Out"=w225:refnum<class "Scope5761.lvclass">)  [unwired: 8 in, 1 out]
          }
          event "Singleshot": Value Change {
            n158 = event-data() -> ()  [unwired: 1 in, 6 out]
            n159 = local write "Rumode"(FALSE ("Rumode")) -> ()
            n160 = call-dynamic "SetRunMode.vi"("RunMode"=ScopeMode."Single" ("scope mode"), "ScopeBase in"=w230) -> ("ScopeBase out"=w228:refnum<class "Scope5761.lvclass">)  [unwired: 8 in, 1 out]
          }
          event "Rumode": Value Change {
            n161 = event-data() -> ()  [unwired: 1 in, 6 out]
            n162 = case shown="\"Triggered\"" "Trigmode" {
              tunnel: [ScopeMode."Running" ("scope mode") ScopeMode."Continuous" ("scope mode")] -> w235
              frame "Triggered" {
              }
              frame "Continuous" {
              }
            }
            n163 = Select(t=w235, s="Rumode", f=ScopeMode."Stopped" ("scope mode")) -> (s? t:f=w233:T14)
            n164 = call-dynamic "SetRunMode.vi"("RunMode"=w233, "ScopeBase in"=w234) -> ("ScopeBase out"=w232:refnum<class "Scope5761.lvclass">)  [unwired: 8 in, 1 out]
          }
          event Value Change {
            n165 = event-data() -> ("CtlRef"=w243:refnum<vi>, "NewVal"=w241:bool)  [unwired: 1 in, 4 out]
            n166 = Search 1D Array(1D array=w244, element=w243) -> (index of element=w242:i32)  [unwired: 1 in]
            n167 = property on="Upper chart" class="WFChart (strict)"("Active Plot"=w242, "Plot.Visible?"=w241) -> ()  [unwired: 2 in, 2 out]
          }
          event Value Change {
            n168 = event-data() -> ("CtlRef"=w249:refnum<vi>, "NewVal"=w246:bool)  [unwired: 1 in, 4 out]
            n169 = Search 1D Array(1D array=w248, element=w249) -> (index of element=w247:i32)  [unwired: 1 in]
            n170 = property on="freqdata" class="WFGraph (strict)"("Active Plot"=w247, "Plot.Visible?"=w246) -> ()  [unwired: 2 in, 2 out]
            n171 = property on="Lower chart" class="WFChart (strict)"("Active Plot"=w247, "Plot.Visible?"=w246) -> ()  [unwired: 2 in, 2 out]
          }
          event "stop": Value Change {
            n172 = event-data() -> ()  [unwired: 1 in, 6 out]
          }
          event Value Change {
            n173 = event-data() -> ()  [unwired: 1 in, 6 out]
            n174 = case shown="\"V\"" "Unit" {
              tunnel: ["V" "dBV" "V^2"] -> w255
              frame "V" {
              }
              frame "dBV" {
              }
              frame "V^2" {
              }
            }
            n175 = Concatenate Strings("Amplitude [", w255, "]") -> (w253:string)
            n176 = property on="freqdata" class="WFGraph (strict)"("YScale.NameLbl.Text"=w253) -> ()  [unwired: 2 in, 2 out]
          }
          event "#bins": Value Change {
            n177 = event-data() -> ()  [unwired: 1 in, 6 out]
            n178 = local read "Upper chart"() -> (w264:dbl[][])
            n179 = local read "Window"() -> (w265:T9)
            n180 = local read "Unit"() -> (w266:T8)
            n181 = call "calc FFT.vi"("#bins"="#bins", "dt"=1e-06, "Unit"=w266, "Window"=w265, "data"=w264) -> ("Power Spectrum / PSD"=w263:cluster{"f0":dbl, "df":dbl, "magnitude":dbl[]}[])  [unwired: 6 in]
            n182 = local write "freqdata"(w263) -> ()
          }
          event "Zoom time X", "Zoom time Y": Value Change {
            n183 = event-data() -> ()  [unwired: 1 in, 6 out]
            n184 = control-ref of="Upper chart"() -> (w271:refnum<vi>)
            n185 = call "setZoomTool.vi"("Zoom Y"="Zoom time Y", "Zoom  X"="Zoom time X", "reference"=w271) -> ()  [unwired: 9 in]
            n186 = call "setZoomTool.vi"("Zoom Y"="Zoom time Y", "Zoom  X"="Zoom time X") -> ()  [unwired: 10 in]
          }
          event "Zoom freq Y", "Zoom freq X": Value Change {
            n187 = event-data() -> ()  [unwired: 1 in, 6 out]
            n188 = control-ref of="Lower chart"() -> (w276:refnum<vi>)
            n189 = control-ref of="Lower graph"() -> (w275:refnum<vi>)
            n190 = control-ref of="freqdata"() -> (w277:refnum<vi>)
            n191 = call "setZoomTool.vi"("Zoom Y"="Zoom freq Y", "Zoom  X"="Zoom freq X", "reference"=w277) -> ()  [unwired: 9 in]
            n192 = call "setZoomTool.vi"("Zoom Y"="Zoom freq Y", "Zoom  X"="Zoom freq X", "reference"=w276) -> ()  [unwired: 9 in]
            n193 = call "setZoomTool.vi"("Zoom Y"="Zoom freq Y", "Zoom  X"="Zoom freq X", "reference"=w275) -> ()  [unwired: 9 in]
          }
          event Value Change {
            w287 = dbl[][] [] ("History Data")
            n194 = event-data() -> ()  [unwired: 1 in, 6 out]
            n195 = case shown="\"Time and Frequency\", Default" "Display" {
              tunnel: ["deltaF" _] -> w282
              frame "Time and Frequency", Default {
              }
              frame "Phase and Magnitude" {
              }
            }
            n196 = property on="Upper chart" class="WFChart (strict)"("History Data"=w287) -> ()  [unwired: 2 in, 2 out]
            n197 = property on="Lower chart" class="WFChart (strict)"("History Data"=w287) -> ()  [unwired: 2 in, 2 out]
            n198 = local write "freqdata"(cluster{"f0":dbl, "df":dbl, "magnitude":dbl[]}[] [] ("freqdata")) -> ()
            n199 = call "UpdateGraphs.vi"("Buffer mode"="Buffer", "Display mode"="Display", "Graph_refs"=w288) -> ()  [unwired: 9 in]
            n200 = property on="Zoom time X" class="Bool (strict)"("Val(Sgnl)"=TRUE ("Value (Signaling)")) -> ()  [unwired: 2 in, 2 out]
            n201 = property on="Upper chart" class="WFChart (strict)"("Active Plot"=u32 3, "Plot.Visible?"=w282) -> ()  [unwired: 2 in, 2 out]
            n202 = call "Write last phase.vi"("last phase"=dbl[] [0.0, 0.0], "ScopeBase in"=w281) -> ("ScopeBase out"=w279:refnum<class "Scope5761.lvclass">)  [unwired: 8 in, 1 out]
          }
        }
      }
      "stop 2" <- w106
    }
    frame Error {
    }
  }
  n203 = Unregister For Events(event registration refnum=w86) -> ()  [unwired: 1 in, 1 out]
  n204 = flat-sequence {
    tunnel: w1 -> [w293]
    frame #0 {
      n205 = call-dynamic "Close.vi"("ScopeBase in"=w293) -> ()  [unwired: 11 in]
      n206 = global write "global_stop.vi" "Stop"(TRUE ("Stop")) -> ()
    }
  }
